vi "ContrlJudgeStopMove.vi"() -> (1 "是否停止运动？":bool)   [LabVIEW 2018]
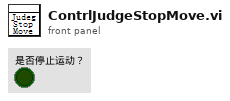
[diagram p1: front panel]
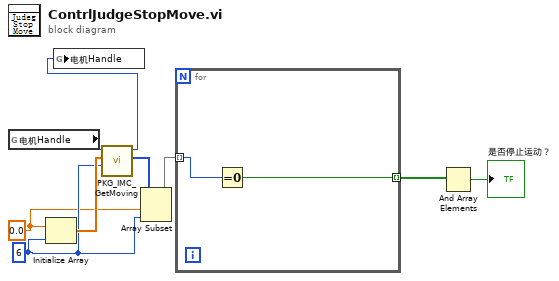
[diagram p0: block diagram]
diagram:
  w4 = 6 ("维数大小")
  w3 = 0.0 ("元素")
  n1 = global read "参数.vi" "电机Handle"() -> (w9:u32)
  n2 = Initialize Array(w3, w4) -> (w8:dbl[])
  n3 = call "PKG_IMC_GetMoving.vi"("axisnum"=w4, "moving"=w8, "Handle"=w9) -> ("moving out"=w5:u16[], "Handle out"=w1:u32)  [unwired: 6 in, 1 out]
  n4 = global write "参数.vi" "电机Handle"(w1) -> ()
  n5 = Array Subset(array=w5, index=w3, length=w4) -> (w2:u16[])
  n6 = for {
    tunnel: w2 -> [w11] mode=indexing
    tunnel: [w10] -> w7 mode=indexing
    n7 = Equal To 0?(x=w11) -> (x = 0?=w10:bool)
  }
  n8 = And Array Elements(Boolean array=w7) -> (logical AND=→"是否停止运动？":bool)
